vi "scaninput.vi"(8 "error in (no error)":errorcluster, 11 "2410C-64 in":refnum<class "2410C-64.lvclass">) -> (0 "error out":errorcluster, 3 "2410C-64 out":refnum<class "2410C-64.lvclass">)   [LabVIEW 2019, in "2410C-64.lvclass"]
uses:
  2410C-64.lvclass
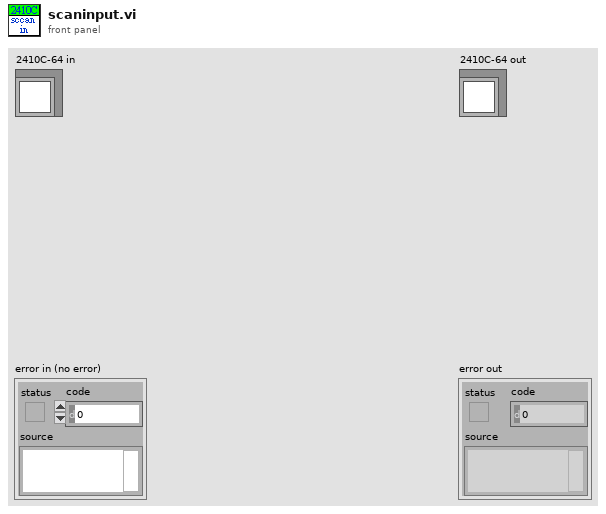
[diagram p1: front panel]
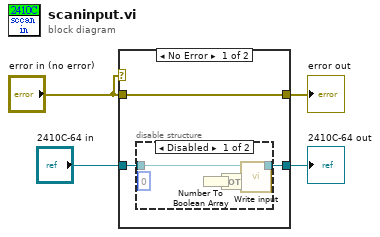
[diagram p0: block diagram]
diagram:
  n1 = case shown="No Error" "error in (no error)" {
    tunnel: [w7 w13] -> w4
    tunnel: "error in (no error)" -> [w7 w13]
    tunnel: "2410C-64 in" -> [w6 w14]
    tunnel: [w5 w14] -> w1
    frame No Error {
      n2 = disable-structure shown="Disabled" {
        disable-tunnel: w6 -> [w11 w12]
        disable-tunnel: [w10 w12] -> w5
        frame Disabled {
          (unwired) u16 0 ("cardno")
          n3 = Number To Boolean Array() -> (Boolean array=w9:bool[])  [unwired: 1 in]
          n4 = Not(x=w9) -> (.not. x?=w8:bool[])
          n5 = call-dynamic "Write input.vi"("input"=w8, "IOCard in"=w11) -> ("IOCard out"=w10:refnum<class "2410C-64.lvclass">)  [unwired: 8 in, 1 out]
        }
        frame Enabled {
        }
      }
    }
    frame Error {
    }
  }
  "error out" <- w4
  "2410C-64 out" <- w1
